vi "PostCopyScripting.vi"(10 "MetaDataObj":refnum<class "MetaDataObj.lvclass">, 11 "User Project":refnum<vi>) -> ()   [LabVIEW 2013, in "UserTBModuleDecideFeatures.lvclass"]
uses:
  UserTBModuleDecideFeatures.lvclass
  <resource>/dialog/NewProjectWizard/MetaDataObj/MetaDataObj.lvclass
  UserTBModuleDecideFeatures.lvclass/UserTBModuleDecideFeatures.ctl
  Read component name.vi
  <vilib>/Utility/EditLVLibs/Edit LVLibs.lvlib
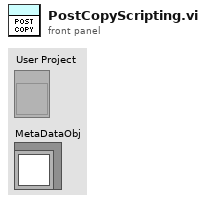
[diagram p1: front panel]
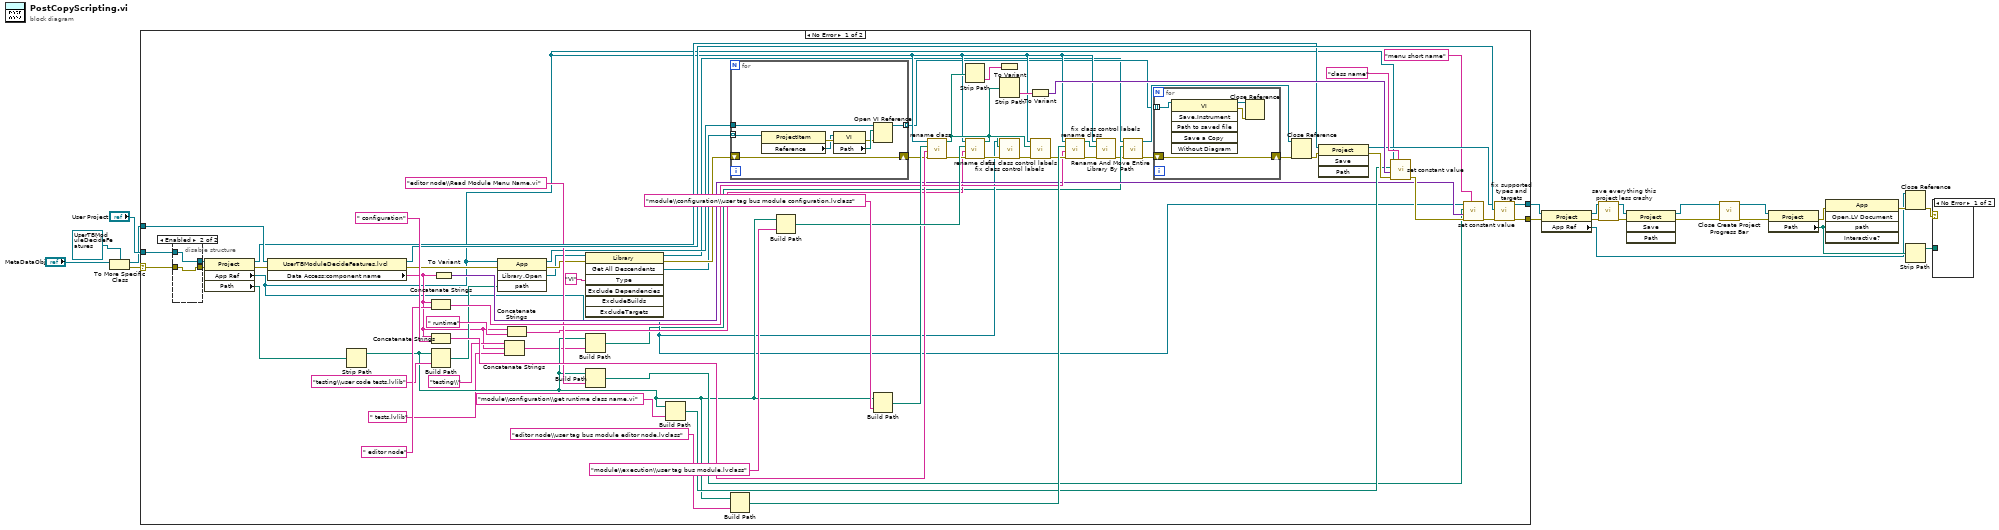
[diagram p0: block diagram]
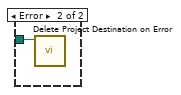
[diagram p2: hidden frame]
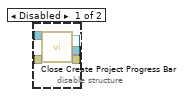
[diagram p3: hidden frame]
diagram:
  n1 = To More Specific Class(target class=refnum<class "UserTBModuleDecideFeatures.lvclass"> refnum ("DecideProjectFeatures.lvclass"), reference="MetaDataObj") -> (specific class reference=w14:refnum<class "UserTBModuleDecideFeatures.lvclass">, error out=w19:errorcluster)  [unwired: 1 in]
  n2 = case shown="No Error" w19 {
    selector: w19 -> [w72 w109]
    tunnel: [w60 w110] -> w11
    tunnel: "User Project" -> [w71 w110]
    tunnel: [w61 w109] -> w10
    tunnel: w14 -> [w86 _]
    frame No Error {
      n3 = disable-structure shown="Enabled" {
        disable-tunnel: w72 -> [w94 w95]
        disable-tunnel: w71 -> [w93 w96]
        disable-tunnel: [w92 w96] -> w70
        disable-tunnel: [w91 w95] -> w69
        frame Disabled {
          n4 = call <resource>:"Close Create Project Progress Bar.vi"("error in (no error)"=w94, "Project"=w93) -> ("error out"=w91:errorcluster, "dup Project"=w92:refnum<vi>)  [unwired: 8 in]
        }
        frame Enabled {
        }
      }
      n5 = property class="Project"(reference=w70, error in=w69) -> (reference out=w76:refnum<vi>, error out=w90:errorcluster, "App Ref"=w31:refnum<vi>, "Path"=w89:path)
      n6 = property class="UserTBModuleDecideFeatures.lvcl"(reference=w86, error in=w90) -> (reference out=w81:refnum<class "UserTBModuleDecideFeatures.lvclass">, error out=w39:errorcluster, "Data Access:component name"=w32:string)
      n7 = Strip Path(path=w89) -> (stripped path=w36:path)  [unwired: 1 out]
      n8 = Concatenate Strings(w32, " editor node" ("string")) -> (w62:string)
      n9 = Concatenate Strings(w32, " configuration" ("string")) -> (w58:string)
      n10 = Build Path(base path=w36, name or relative path="testing\\user code tests.lvlib") -> (appended path=w37:path)
      n11 = To Variant(anything=w32) -> (Variant=w50:variant)
      n12 = invoke class="App" method="Library.Open"(reference=w31, error in=w39, "path"=w37) -> (reference out=w41:refnum<vi>, error out=w45:errorcluster, "Open Library"=w44:refnum<vi>)  [unwired: 1 in, 1 out]
      n13 = Concatenate Strings("testing\\" ("string"), w32, " tests.lvlib" ("string")) -> (w34:string)
      n14 = Concatenate Strings(w32, " runtime" ("string")) -> (w46:string)
      n15 = invoke class="Library" method="Get All Descendents"(reference=w44, error in=w45, "Type"="VI") -> (reference out=w24:refnum<vi>, error out=w42:errorcluster, "All Descendents"=w25:refnum<vi>[])  [unwired: 4 in, 4 out]
      n16 = Build Path(base path=w36, name or relative path=w34) -> (appended path=w23:path)
      n17 = Build Path(base path=w36, name or relative path="editor node\\Read Module Menu Name.vi") -> (appended path=w48:path)
      n18 = Build Path(base path=w36, name or relative path="module\\configuration\\get runtime class name.vi") -> (appended path=w57:path)
      n19 = for {
        tunnel: [w104] -> w27 mode=indexing
        shift-right: [w103] -> w40
        shift-left: w42 -> [w103]
        tunnel: w41 -> [w102]
        tunnel: w25 -> [w101] mode=indexing
        n20 = property class="ProjectItem"(reference=w101) -> (error out=w108:errorcluster, "Reference"=w107:refnum<vi>)  [unwired: 1 in, 1 out]
        n21 = property class="VI"(reference=w107, error in=w108) -> (error out=w105:errorcluster, "Path"=w106:path)  [unwired: 1 out]
        n22 = Open VI Reference(application reference (local)=w102, vi path=w106, error in (no error)=w105) -> (vi reference=w104:refnum<vi>)  [unwired: 3 in, 1 out]
      }
      n23 = Build Path(base path=w36, name or relative path="editor node\\user tag bus module editor node.lvclass") -> (appended path=w67:path)
      n24 = Build Path(base path=w36, name or relative path="module\\execution\\user tag bus module.lvclass") -> (appended path=w85:path)
      n25 = Build Path(base path=w36, name or relative path="module\\configuration\\user tag bus module configuration.lvclass") -> (appended path=w82:path)
      n26 = call "rename class.vi"("error in"=w40, "new name"=w58, "class path"=w82, "Application in"=w31) -> ("error out"=w83:errorcluster, "New Library Path"=w53:path)  [unwired: 6 in]
      n27 = Strip Path(path=w53) -> (name=w54:string)  [unwired: 1 out]
      n28 = call "rename class.vi"("error in"=w83, "new name"=w46, "class path"=w85, "Application in"=w31) -> ("error out"=w74:errorcluster, "New Library Path"=w55:path)  [unwired: 6 in]
      n29 = To Variant(anything=w54) -> ()  [unwired: 1 out]
      n30 = Strip Path(path=w55) -> (name=w56:string)  [unwired: 1 out]
      n31 = call "fix class control labels.vi"("error in"=w74, "class to load"=w53, "Application in"=w31) -> ("error out"=w73:errorcluster)  [unwired: 8 in]
      n32 = To Variant(anything=w56) -> (Variant=w80:variant)
      n33 = call "fix class control labels.vi"("error in"=w73, "class to load"=w55, "Application in"=w31) -> ("error out"=w64:errorcluster)  [unwired: 8 in]
      n34 = call "rename class.vi"("error in"=w64, "new name"=w62, "class path"=w67, "Application in"=w31) -> ("error out"=w65:errorcluster, "New Library Path"=w66:path)  [unwired: 6 in]
      n35 = call "fix class control labels.vi"("error in"=w65, "class to load"=w66, "Application in"=w31) -> ("error out"=w22:errorcluster)  [unwired: 8 in]
      n36 = call <vilib>:"Rename And Move Entire Library By Path.vi"("error in (no error)"=w22, "New library path"=w23, "Library ref in"=w24) -> ("error out"=w29:errorcluster, "Library ref out"=w30:refnum<vi>)  [unwired: 7 in]
      n37 = for {
        tunnel: w27 -> [w100] mode=indexing
        shift-right: [w97] -> w28
        shift-left: w29 -> [w97]
        n38 = invoke class="VI" method="Save.Instrument"(reference=w100) -> (reference out=w98:refnum<vi>, error out=w99:errorcluster)  [unwired: 5 in, 4 out]
        n39 = Close Reference(reference=w98, error in (no error)=w99) -> ()  [unwired: 1 out]
      }
      n40 = Close Reference(reference=w30, error in (no error)=w28) -> (error out=w26:errorcluster)
      n41 = invoke class="Project" method="Save"(reference=w76, error in=w26) -> (reference out=w75:refnum<vi>, error out=w77:errorcluster)  [unwired: 2 in, 2 out]
      n42 = call "set constant value.vi"("control name"="class name", "error in"=w77, "data to set"=w80, "vi path"=w57, "Application in"=w31) -> ("error out"=w59:errorcluster)  [unwired: 6 in]
      n43 = call "set constant value.vi"("control name"="menu short name", "error in"=w59, "data to set"=w50, "vi path"=w48, "Application in"=w31) -> ("error out"=w52:errorcluster)  [unwired: 6 in]
      n44 = call "fix supported types and targets.vi"("error in"=w52, "DecideProjectFeatures in"=w81, "User Project in"=w75) -> ("error out"=w61:errorcluster, "User Project out"=w60:refnum<vi>)  [unwired: 7 in]
    }
    frame Error {
    }
  }
  n45 = property class="Project"(reference=w11, error in=w10) -> (reference out=w8:refnum<vi>, error out=w9:errorcluster, "App Ref"=w7:refnum<vi>)
  n46 = call "save everything this project less crashy.vi"("error in"=w9, "Project in"=w8) -> ("error out"=w13:errorcluster, "Project out"=w12:refnum<vi>)  [unwired: 8 in]
  n47 = invoke class="Project" method="Save"(reference=w12, error in=w13) -> (reference out=w1:refnum<vi>, error out=w4:errorcluster)  [unwired: 2 in, 2 out]
  n48 = call <resource>:"Close Create Project Progress Bar.vi"("error in (no error)"=w4, "Project"=w1) -> ("error out"=w2:errorcluster, "dup Project"=w3:refnum<vi>)  [unwired: 8 in]
  n49 = property class="Project"(reference=w3, error in=w2) -> (error out=w18:errorcluster, "Path"=w15:path)  [unwired: 1 out]
  n50 = invoke class="App" method="Open.LV Document"(error in=w18, "path"=w15) -> (error out=w17:errorcluster)  [unwired: 3 in, 4 out]
  n51 = Close Reference(reference=w7, error in (no error)=w17) -> (error out=w6:errorcluster)
  n52 = Strip Path(path=w15) -> (stripped path=w5:path)  [unwired: 1 out]
  n53 = case shown="No Error" w6 {
    tunnel: w5 -> [_ w111]
    frame No Error {
    }
    frame Error {
      n54 = call <resource>:"Delete Project Destination on Error.vi"("Project Destination Root"=w111) -> ()  [unwired: 11 in]
    }
  }
